vi "Event Stuffer.vi"() -> ()   [LabVIEW 2009, in "Database.lvlib"]
uses:
  Database.lvlib
  interface/Pelletron.ctl
  interface/Dust Info.ctl
  interface/Timetrace.ctl
  interface/Data Source.ctl
  interface/Dust Head.ctl
  Dust Event.ctl
  interface/Interface.lvlib
  Data Store.lvclass
  waveform/Waveform.lvlib
panel:
  out "Last Event Posted to Database":T1
  out "Dust Head update status":bool
  out "Dust Head Error":errorcluster
  out "Dust Head Iterations":i32
  out "Dust Head":T2
  out "Dust Iterations":i32
  out "# elements in queue":i32
  out "Pelletron iterations":i32
  out "Dust Event Error":errorcluster
  out "Pelletron Error":errorcluster
  in  "stop":bool
  out "Pelletron update status":bool
  out "Last HDF5 File Written":string
  out "Last Dust Trace":T3
  out "Last Pelletron Tick":T6
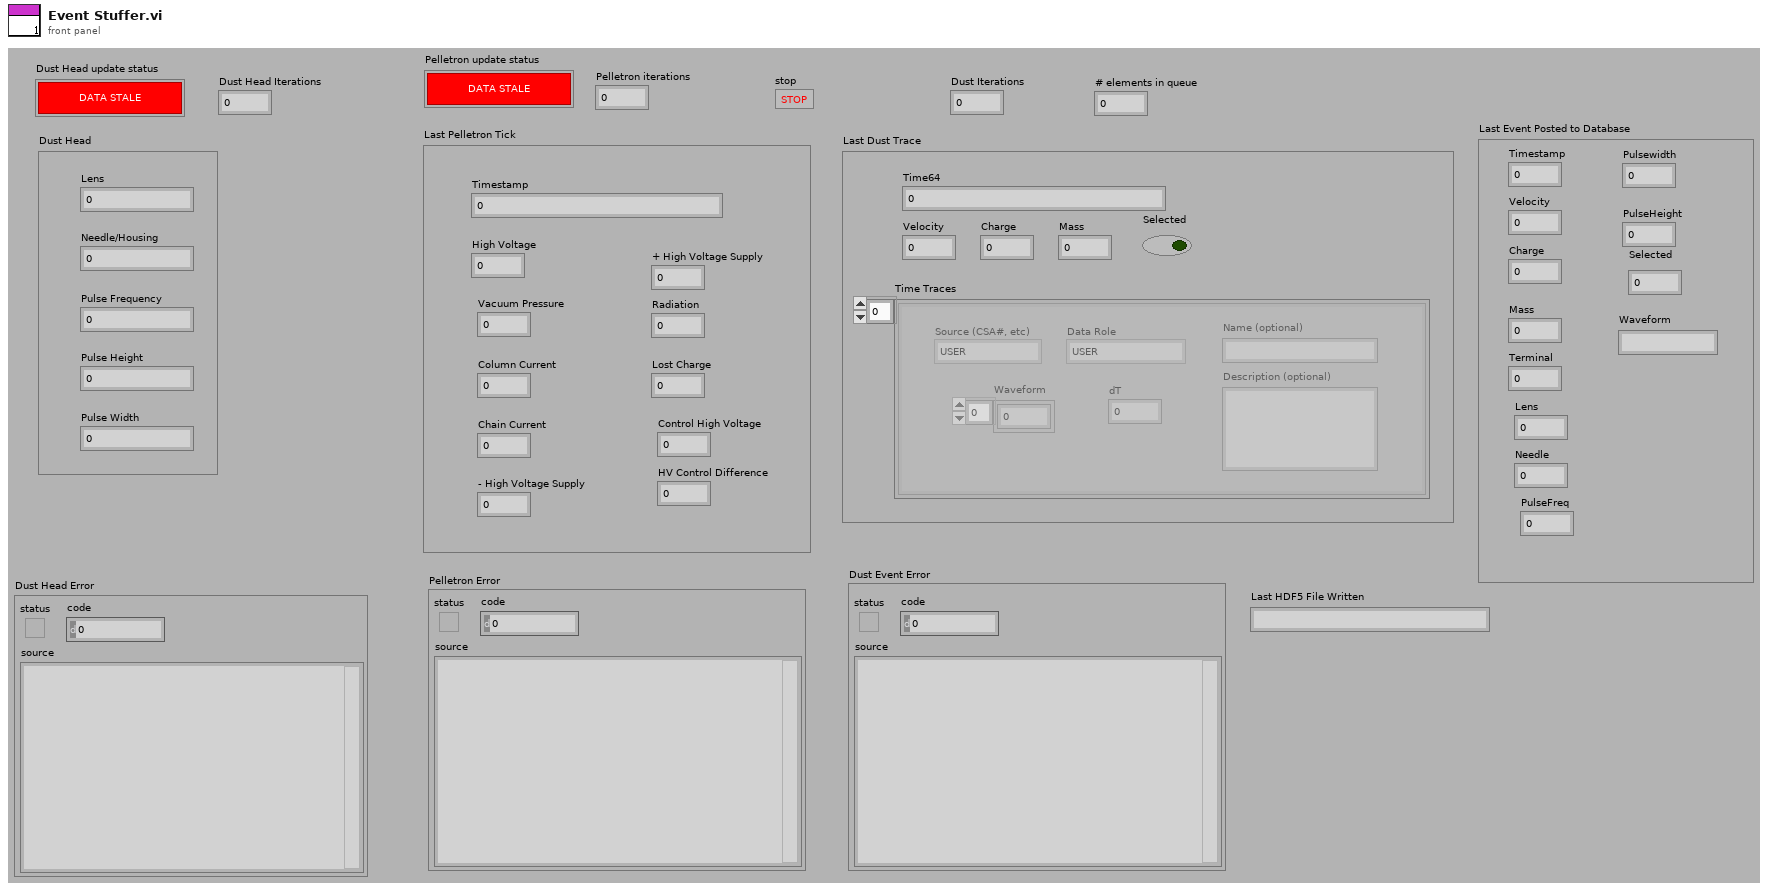
[diagram p1: front panel]
types:
  T1 = typedef "Database.lvlib/Dust Event.ctl" = cluster{"Timestamp":u64, "Velocity":sgl, "Charge":sgl, "Mass":sgl, "Terminal":sgl, "Lens":sgl, "Needle":sgl, "PulseFreq":sgl, "Pulsewidth":dbl, "PulseHeight":sgl, "Selected":i8, "Waveform":string}
  T2 = typedef "Interface.lvlib/Dust Head.ctl" = cluster{"Lens":dbl, "Needle/Housing":dbl, "Pulse Frequency":dbl, "Pulse Height":dbl, "Pulse Width":dbl}
  T3 = typedef "Interface.lvlib/Dust Info.ctl" = cluster{"Time64":u64, "Velocity":dbl, "Charge":dbl, "Mass":dbl, "Time Traces":T4[], "Selected":bool}
  T4 = typedef "Interface.lvlib/Timetrace.ctl" = cluster{"Source (CSA#, etc)":T5, "Data Role":enum16{"USER", "FIRST DETECTOR", "SECOND DETECTOR", "THIRD DETECTOR", "FINAL DETECTOR"}, "Waveform":sgl[], "dT":sgl, "Name (optional)":string, "Description (optional)":string}
  T5 = typedef "Interface.lvlib/Data Source.ctl" = enum16{"USER", "CSA1", "CSA2", "CSA3", "CSA4", "CSA5", "CSA6", ""}
  T6 = typedef "Interface.lvlib/Pelletron.ctl" = cluster{"Timestamp":u64, "High Voltage":sgl, "Vacuum Pressure":sgl, "Column Current":sgl, "Chain Current":sgl, "- High Voltage Supply":dbl, "+ High Voltage Supply":dbl, "Radiation":dbl, "Lost Charge":dbl, "Control High Voltage":dbl, "HV Control Difference":dbl}
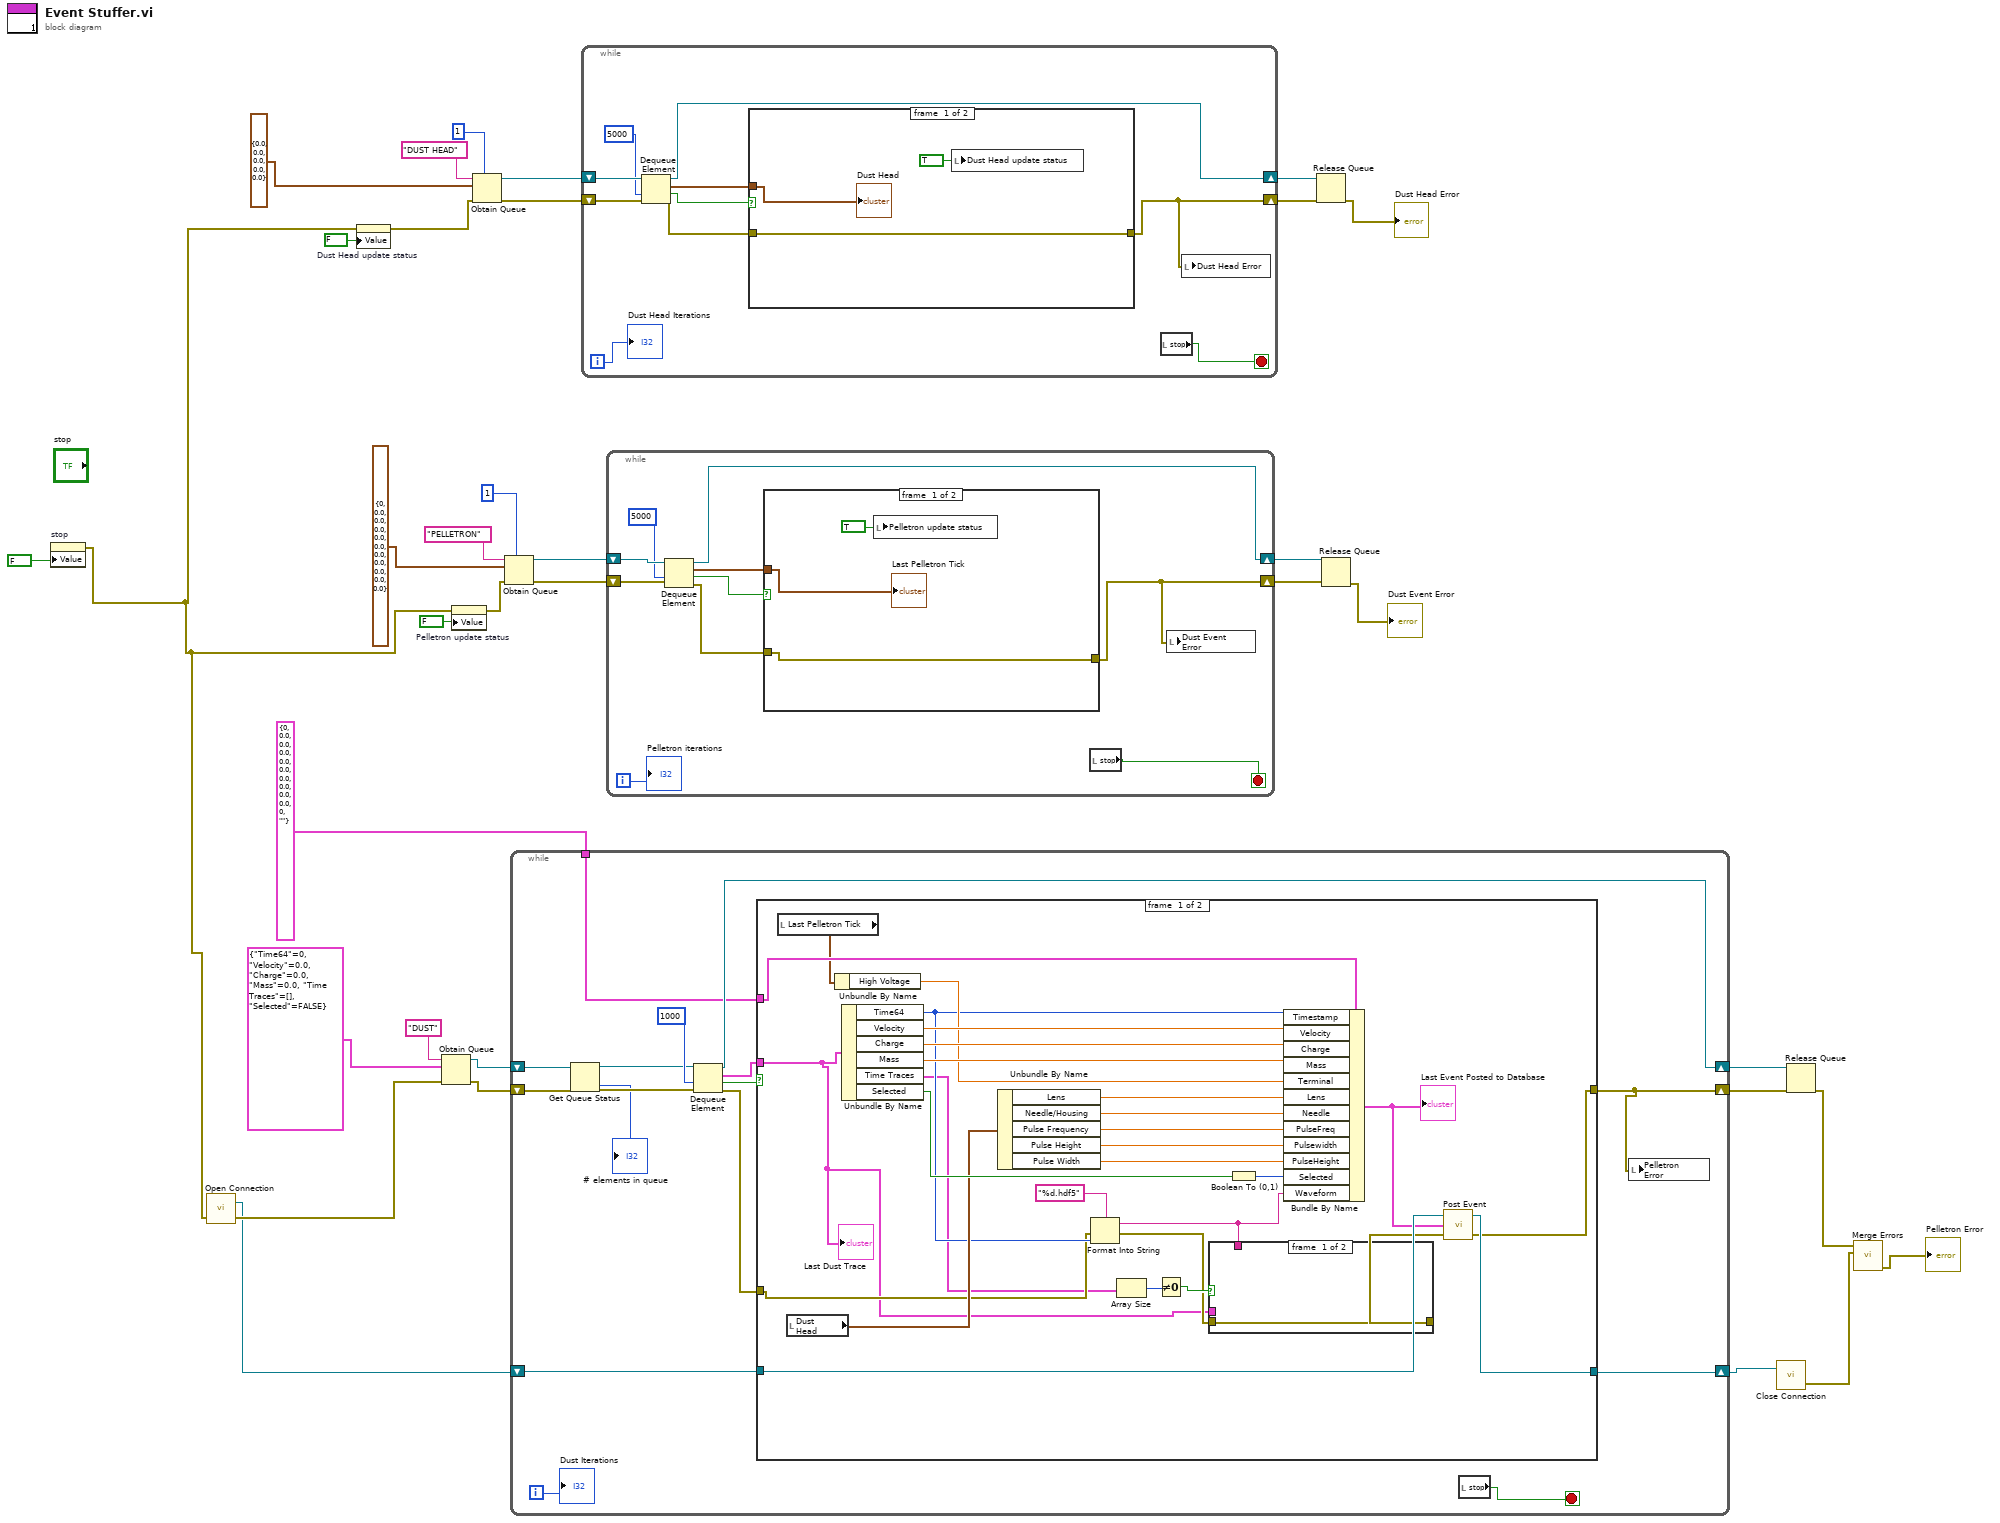
[diagram p0: block diagram]
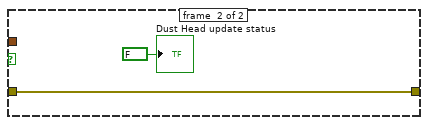
[diagram p2: hidden frame]
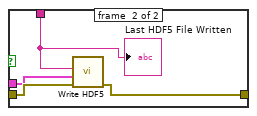
[diagram p3: hidden frame]
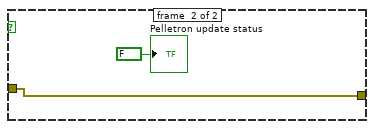
[diagram p5: hidden frame]
diagram:
  n1 = property on="stop" class="Bool (strict)"("Value"=FALSE) -> (error out=w7:errorcluster)  [unwired: 2 in, 1 out]
  n2 = call "Open Connection.vi"("error in (no error)"=w7) -> ("error out"=w6:errorcluster, "Database.lvlib:Data Store.lvclass"=w5:refnum<class "Data Store.lvclass">)  [unwired: 1 in]
  n3 = property on="Dust Head update status" class="Bool (strict)"(error in=w7, "Value"=FALSE ("Dust Head update status")) -> (error out=w15:errorcluster)  [unwired: 1 in, 1 out]
  n4 = Obtain Queue(name (unnamed)="DUST", element data type=T3 {"Time64"=0, "Velocity"=0.0, "Charge"=0.0, "Mass"=0.0, "Time Traces"=[], "Selected"=FALSE} ("Cluster"), error in (no error)=w6) -> (queue out=w23:refnum<queue>, error out=w22:errorcluster)  [unwired: 2 in, 1 out]
  n5 = property on="Pelletron update status" class="Bool (strict)"(error in=w7, "Value"=FALSE ("Pelletron update status")) -> (error out=w28:errorcluster)  [unwired: 1 in, 1 out]
  n6 = Obtain Queue(max queue size (-1, unlimited)=1, name (unnamed)="DUST HEAD", element data type=T2 {"Lens"=0.0, "Needle/Housing"=0.0, "Pulse Frequency"=0.0, "Pulse Height"=0.0, "Pulse Width"=0.0} ("Cluster"), error in (no error)=w15) -> (queue out=w16:refnum<queue>, error out=w17:errorcluster)  [unwired: 1 in, 1 out]
  n7 = Obtain Queue(max queue size (-1, unlimited)=1, name (unnamed)="PELLETRON", element data type=T6 {"Timestamp"=0, "High Voltage"=0.0, "Vacuum Pressure"=0.0, "Column Current"=0.0, "Chain Current"=0.0, "- High Voltage Supply"=0.0, "+ High Voltage Supply"=0.0, "Radiation"=0.0, "Lost Charge"=0.0, "Control High Voltage"=0.0, "HV Control Difference"=0.0} ("Cluster"), error in (no error)=w28) -> (queue out=w33:refnum<queue>, error out=w32:errorcluster)  [unwired: 1 in, 1 out]
  n8 = while {
    shift-right: [w42] -> w9
    shift-left: w23 -> [w48]
    shift-right: [w38] -> w8
    shift-left: w22 -> [w46]
    tunnel: T1 {"Timestamp"=0, "Velocity"=0.0, "Charge"=0.0, "Mass"=0.0, "Terminal"=0.0, "Lens"=0.0, "Needle"=0.0, "PulseFreq"=0.0, "Pulsewidth"=0.0, "PulseHeight"=0.0, "Selected"=0, "Waveform"=""} ("Cluster") -> [w40]
    shift-right: [w36] -> w4
    shift-left: w5 -> [w37]
    i -> [w43]
    stop <- w39 stop-if-true
    n9 = Get Queue Status(queue=w48, error in (no error)=w46) -> (queue out=w47:refnum<queue>, error out=w45:errorcluster, # elements in queue=→"# elements in queue":i32)  [unwired: 1 in, 5 out]
    n10 = Dequeue Element(queue=w47, timeout in ms (-1)=1000, error in (no error)=w45) -> (queue out=w42:refnum<queue>, element=w41:T3, timed out?=w50:bool, error out=w49:errorcluster)
    n11 = case shown="False" w50 {
      tunnel: w49 -> [w63 w86]
      tunnel: [w59 w86] -> w38
      tunnel: w41 -> [w53 _]
      tunnel: w40 -> [w79 _]
      tunnel: w37 -> [w62 w85]
      tunnel: [w60 w85] -> w36
      frame #0 {
        n12 = local read "Last Pelletron Tick"() -> (w75:T6)
        n13 = local read "Dust Head"() -> (w71:T2)
        n14 = Unbundle By Name(w75) -> ("High Voltage"=w74:sgl)
        n15 = Unbundle By Name(w53) -> ("Time64"=w64:u64, "Velocity"=w78:dbl, "Charge"=w77:dbl, "Mass"=w76:dbl, "Time Traces"=w55:T4[], "Selected"=w73:bool)
        n16 = Unbundle By Name(w71) -> ("Lens"=w70:dbl, "Needle/Housing"=w69:dbl, "Pulse Frequency"=w68:dbl, "Pulse Height"=w67:dbl, "Pulse Width"=w66:dbl)
        n17 = Format Into String(format string="%d.hdf5", error in=w63, w64) -> (resulting string=w54:string, error out=w56:errorcluster)  [unwired: 1 in]
        n18 = Array Size(array=w55) -> (size(s)=w58:i32)
        n19 = Not Equal To 0?(x=w58) -> (x != 0?=w57:bool)
        n20 = case shown="True" w57 {
          tunnel: w56 -> [w80 w84]
          tunnel: w53 -> [_ w82]
          tunnel: [w80 w83] -> w52
          tunnel: w54 -> [_ w81]
          frame #0 {
          }
          frame #1 {
            n21 = call "Write HDF5.vi"("error in (no error)"=w84, "Cluster"=w82, "Filename"=w81) -> ("error out"=w83:errorcluster)  [unwired: 8 in]
            "Last HDF5 File Written" <- w81
          }
        }
        n22 = Boolean To (0,1)(Boolean=w73) -> (0, 1=w72:i16)
        n23 = Bundle By Name(cluster=w79, "Timestamp"=w64, "Velocity"=w78, "Charge"=w77, "Mass"=w76, "Terminal"=w74, "Lens"=w70, "Needle"=w69, "PulseFreq"=w68, "Pulsewidth"=w67, "PulseHeight"=w66, "Selected"=w72, "Waveform"=w54) -> (w61:T1)
        "Last Event Posted to Database" <- w61
        n24 = call "Post Event.vi"("error in (no error)"=w52, "Event In"=w61, "Database.lvlib:Data Store.lvclass"=w62) -> ("error out"=w59:errorcluster, "Database.lvlib:Data Store.lvclass 2"=w60:refnum<class "Data Store.lvclass">)  [unwired: 1 in]
        "Last Dust Trace" <- w53
      }
      frame #1 {
      }
    }
    n25 = local read "stop"() -> (w39:bool)
    n26 = local write "Pelletron Error"(w38) -> ()
    "Dust Iterations" <- w43
  }
  n27 = while {
    shift-right: [w90] -> w13
    shift-left: w16 -> [w95]
    shift-right: [w88] -> w12
    shift-left: w17 -> [w96]
    i -> [w89]
    stop <- w87 stop-if-true
    n28 = Dequeue Element(queue=w95, timeout in ms (-1)=5000, error in (no error)=w96) -> (queue out=w90:refnum<queue>, element=w91:T2, timed out?=w93:bool, error out=w92:errorcluster)
    n29 = case shown="False" w93 {
      tunnel: w92 -> [w97 w100]
      tunnel: [w97 w100] -> w88
      tunnel: w91 -> [w99 _]
      frame #0 {
        n30 = local write "Dust Head update status"(TRUE ("Dust Head update status")) -> ()
        "Dust Head" <- w99
      }
      frame #1 {
        "Dust Head update status" <- FALSE ("Dust Head update status")
      }
    }
    n31 = local read "stop"() -> (w87:bool)
    n32 = local write "Dust Head Error"(w88) -> ()
    "Dust Head Iterations" <- w89
  }
  n33 = while {
    shift-right: [w106] -> w30
    shift-left: w33 -> [w111]
    shift-right: [w103] -> w31
    shift-left: w32 -> [w109]
    i -> [w104]
    stop <- w102 stop-if-true
    n34 = Dequeue Element(queue=w111, timeout in ms (-1)=5000, error in (no error)=w109) -> (queue out=w106:refnum<queue>, element=w105:T6, timed out?=w107:bool, error out=w108:errorcluster)
    n35 = case shown="False" w107 {
      tunnel: w108 -> [w114 w115]
      tunnel: [w114 w115] -> w103
      tunnel: w105 -> [w113 _]
      frame #0 {
        n36 = local write "Pelletron update status"(TRUE ("Pelletron update status")) -> ()
        "Last Pelletron Tick" <- w113
      }
      frame #1 {
        "Pelletron update status" <- FALSE ("Pelletron update status")
      }
    }
    n37 = local read "stop"() -> (w102:bool)
    n38 = local write "Dust Event Error"(w103) -> ()
    "Pelletron iterations" <- w104
  }
  n39 = Release Queue(queue=w13, error in (no error)=w12) -> (error out=→"Dust Head Error":errorcluster)  [unwired: 1 in, 2 out]
  n40 = Release Queue(queue=w30, error in (no error)=w31) -> (error out=→"Dust Event Error":errorcluster)  [unwired: 1 in, 2 out]
  n41 = call "Close Connection.vi"("Database.lvlib:Data Store.lvclass"=w4) -> ("error out"=w2:errorcluster)  [unwired: 2 in]
  n42 = Release Queue(queue=w9, error in (no error)=w8) -> (error out=w3:errorcluster)  [unwired: 1 in, 2 out]
  n43 = call <vilib>:"Merge Errors.vi"("error in 2 (no error)"=w2, "error in 1 (no error)"=w3) -> ("error out"=→"Pelletron Error":errorcluster)  [unwired: 5 in]
